vi "Log Target.vi"(8 "error in":errorcluster, 10 "Entry":string, 11 "Study Actor in":refnum<class "Study Actor.lvclass">) -> (0 "error out":errorcluster, 3 "Study Actor out":refnum<class "Study Actor.lvclass">)   [LabVIEW 2024, in "Study Actor.lvlib" / "Study Actor.lvclass"]
uses:
  Study Actor.lvclass
  Study Actor.lvclass/Study Actor.ctl
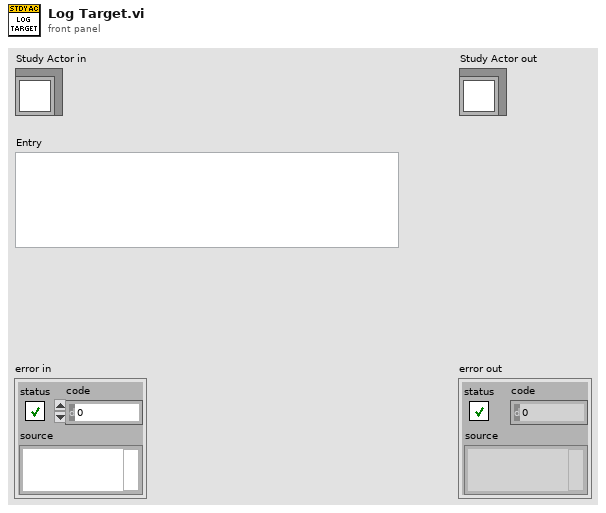
[diagram p1: front panel]
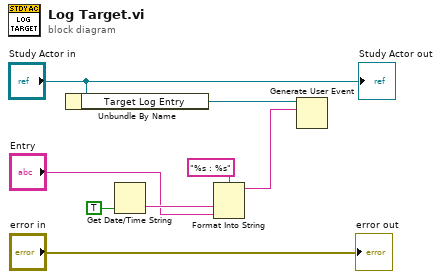
[diagram p0: block diagram]
diagram:
  n1 = Unbundle By Name("Study Actor in") -> ("Target Log Entry"=w2:refnum<user-event>)
  n2 = Get Date/Time String(want seconds? (F)=TRUE) -> (time string=w5:string)  [unwired: 2 in, 1 out]
  n3 = Format Into String(format string="%s : %s", w5, "Entry") -> (resulting string=w1:string)  [unwired: 2 in, 1 out]
  n4 = Generate User Event(user event=w2, event data cluster=w1) -> ()  [unwired: 2 in, 2 out]
  "error out" <- "error in"
  "Study Actor out" <- "Study Actor in"
